vi "IPI_CCD_Base1_X_Cal_Step3.vi"(8 "error in":errorcluster, 9 "Options (Find Straight Edge 1)":T3={"Search Direction"=0, "Edge Options"={"Edge Polarity"=0, "Kernel Size"=5, "Width"=1, "Minimum Edge Strength"=88.0, "Interpolation Type"=enum."Bilinear Fixed", "Data Processing Method"=enum."Average"}, "Show Search Area"=TRUE, "Show Search Lines"=TRUE, "Show Edges Found"=TRUE, "Show Result"=TRUE, "Search Area Color"=65280, "Search Lines Color"=255, "Edge Locations Color"=16776960, "Result Color"=16711680, "Overlay Group Name"=""} {"Search Direction" items=["Left to Right", "Right to Left", "Top to Bottom", "Bottom to Top"]; "Edge Options"."Edge Polarity" items=["All Edges", "Rising Edges", "Falling Edges"]; "Edge Options"."Minimum Edge Strength" format="%.2f"; "Edge Options"."Width" step=2; "Edge Options"."Kernel Size" step=2}, 10 "ROI Descriptor (Find Straight Edge 1)":T6={"Global Rectangle"=[230, 977, 1978, 1125], "Contours"=[{"ID"=enum."External", "Type"=12, "Coordinates"=[230, 977, 1978, 1125, 0]}]} {"Contours"."Type" items=["No Selection", "Point", "Line", "Rectangle", "Oval", "Polygon", "Freehand Region", "Annulus", "Unused2", "Unused3", "Broken Line", "Freehand Line", "Rotated Rectangle"]}, 11 "Image In":T7) -> (0 "error out":errorcluster, 2 "mm":sgl, 3 "Image":T7(plugin-control))   [LabVIEW 2015]
uses:
  <vilib>/vision/Image Controls.llb/IMAQ Image.ctl
  <vilib>/vision/Measure.llb/Straight Edge Options.ctl
  <vilib>/vision/Measure.llb/Straight Edge Process.ctl
  <vilib>/vision/Measure.llb/Edge Options.ctl
  <vilib>/vision/Measure.llb/Edge Polarity.ctl
panel:
  in  "Fit Options (Find Straight Edge 1)":T4={"Number of Lines"=1, "Type"=enum."First Edge Rake", "Min. Score"=10.0, "Max. Score"=1000.0, "Orientation"=0.0, "Angle Range"=45.0, "Angle Tolerance"=1.0, "Step Size"=15, "Min. SNR (db)"=0.0, "Min. Points (%)"=25.0, "Hough Iterations"=5} {"Min. Points (%)" min=0.0 max=100.0; "Min. SNR (db)" min=0.0; "Max. Score" min=0.0 max=1024.0; "Min. Score" min=0.0 max=1024.0 step=1.0}
  in  "ROI Descriptor (Find Straight Edge 1) 2":T6={"Global Rectangle"=[230, 977, 1978, 1125], "Contours"=[{"ID"=enum."External", "Type"=12, "Coordinates"=[230, 977, 1978, 1125, 0]}]} {"Contours"."Type" items=["No Selection", "Point", "Line", "Rectangle", "Oval", "Polygon", "Freehand Region", "Annulus", "Unused2", "Unused3", "Broken Line", "Freehand Line", "Rotated Rectangle"]}
  out "X Distance Piexls":sgl
  out "x-y":cluster{"X":sgl, "Y":sgl}
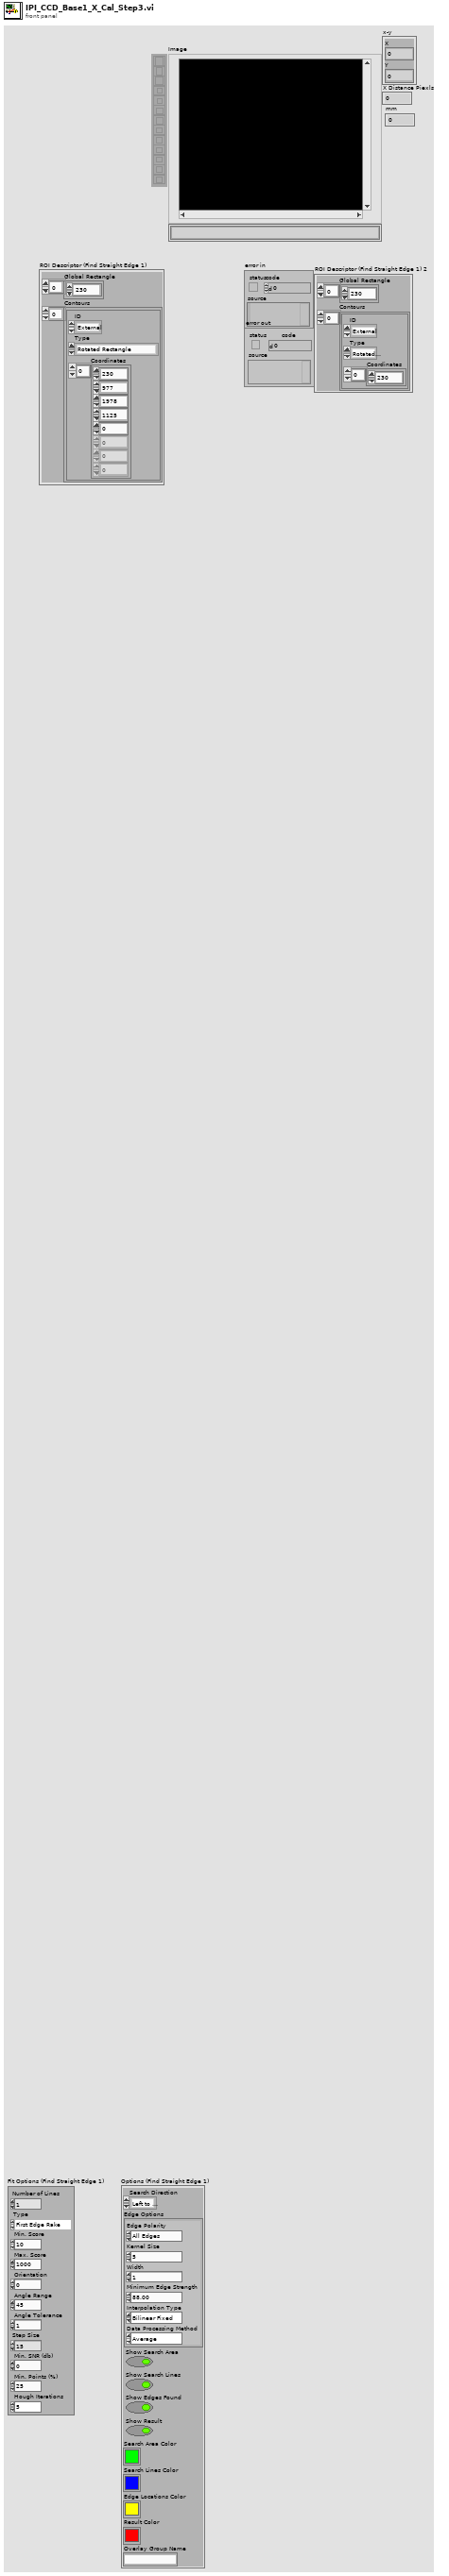
[diagram p1: front panel]
types:
  T1 = typedef "Edge Options.ctl" = cluster{"Edge Polarity":T2, "Kernel Size":u32, "Width":u32, "Minimum Edge Strength":sgl, "Interpolation Type":enum32{"Zero Order", "Bilinear", "Quadratic", "Cubic", "Bilinear Fixed"}, "Data Processing Method":enum32{"Average", "Median"}}
  T2 = typedef "Edge Polarity.ctl" = u32
  T3 = cluster{"Search Direction":u32, "Edge Options":T1, "Show Search Area":bool, "Show Search Lines":bool, "Show Edges Found":bool, "Show Result":bool, "Search Area Color":u32, "Search Lines Color":u32, "Edge Locations Color":u32, "Result Color":u32, "Overlay Group Name":string}
  T4 = typedef "Straight Edge Options.ctl" = cluster{"Number of Lines":i32, "Type":T5, "Min. Score":dbl, "Max. Score":dbl, "Orientation":dbl, "Angle Range":dbl, "Angle Tolerance":dbl, "Step Size":u32, "Min. SNR (db)":dbl, "Min. Points (%)":dbl, "Hough Iterations":i32}
  T5 = typedef "Straight Edge Process.ctl" = enum32{"First Edge Rake", "Best Edge Rake", "Hough Edge Rake", "First Edge Projection", "Best Edge Projection"}
  T6 = cluster{"Global Rectangle":i32[], "Contours":cluster{"ID":enum32{"External", "Internal"}, "Type":u32, "Coordinates":i32[]}[]}
  T7 = typedef "IMAQ Image.ctl" = refnum<image>
  T8 = cluster{"Left":i32, "Top":i32, "Right":i32, "Bottom":i32}
  T9 = cluster{"Point1 (Pixels)":cluster{"X":sgl, "Y":sgl}, "Point2 (Pixels)":cluster{"X":sgl, "Y":sgl}, "Point1 (Real-World)":cluster{"X":sgl, "Y":sgl}, "Point2 (Real-World)":cluster{"X":sgl, "Y":sgl}, "Angle (Pixel)":dbl, "Angle (Real-World)":dbl, "Score":dbl, "Straightness":dbl, "Average SNR (db)":dbl, "Calibration Valid":bool}
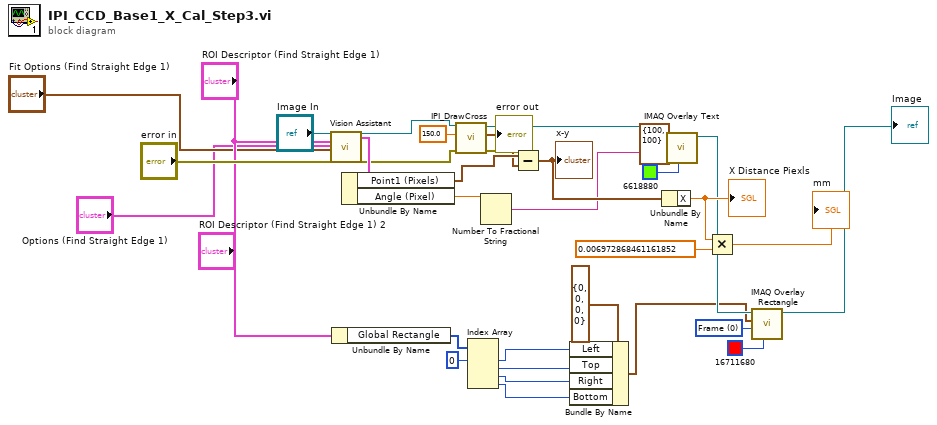
[diagram p0: block diagram]
diagram:
  w13 = u32 0 items=["Frame", "Fill", "Highlight"] ("Drawing Mode (Frame)")
  n1 = call "Vision Assistant"("Image In"="Image In", "ROI Descriptor (Find Straight Edge 1)"="ROI Descriptor (Find Straight Edge 1)", "Options (Find Straight Edge 1)"="Options (Find Straight Edge 1)", "Fit Options (Find Straight Edge 1)"="Fit Options (Find Straight Edge 1)", "error in"="error in") -> ("Image Out"=w32:T7, "Straight Edge (Find Straight Edge 1)"=w31:T9, "error out"=w27:errorcluster)  [unwired: 20 in]
  n2 = Unbundle By Name("ROI Descriptor (Find Straight Edge 1)") -> ("Global Rectangle"=w9:i32[])
  n3 = Unbundle By Name(w31) -> ("Point1 (Pixels)"=w29:cluster{"X":sgl, "Y":sgl}, "Angle (Pixel)"=w19:dbl)
  n4 = call "IPI_DrawCross.vi"("error in (no error)"=w27, "R"=150.0, "Image In"=w32) -> ("error out"=→"error out":errorcluster, "XYCenter"=w28:cluster{"X":i32, "Y":i32}, "Image Out"=w20:T7)  [unwired: 6 in]
  n5 = Index Array(array=w9, index #1=0 ("索引")) -> (element #1=w7:i32, element #2=w6:i32, element #3=w5:i32, element #4=w4:i32)  [unwired: 3 in]
  n6 = Number To Fractional String(number=w19) -> (F-format string=w18:string)  [unwired: 3 in]
  n7 = Subtract(x=w29, y=w28) -> (x-y=w30:cluster{"X":sgl, "Y":sgl})
  "x-y" <- w30
  n8 = Bundle By Name(cluster=T8 {"Left"=0, "Top"=0, "Right"=0, "Bottom"=0} ("Rectangle"), "Left"=w7, "Top"=w6, "Right"=w5, "Bottom"=w4) -> (w3:T8)
  n9 = Unbundle By Name(w30) -> ("X"=w26:sgl)
  "X Distance Piexls" <- w26
  n10 = call "IMAQ Overlay Text"("Text Color (black)"=u32 6618880, "String"=w18, "Origin"=cluster{"X":i32, "Y":i32} {"X"=100, "Y"=100}, "Image"=w20) -> ("Image Out"=w15:T7)  [unwired: 6 in, 1 out]
  n11 = Multiply(x=w26, y=sgl 0.0069728685) -> (x*y=→"mm":sgl)
  n12 = call "IMAQ Overlay Rectangle"("Color"=u32 16711680, "Drawing Mode (Frame)"=w13, "Rectangle"=w3, "Image"=w15) -> ("Image Out"=→"Image":T7)  [unwired: 6 in, 1 out]
